vi "Protocol.Command.Main.vi"(8 "Error":errorcluster, 11 "J1939 Main Configuration":T1 {"Stream Refs"."Port Settings"."FD ISO Mode" items=["ISO", "Non ISO", "ISO Legacy"]; "Stream Refs"."Port Settings"."Termination" items=["Off", "On"]; "Stream Refs"."Port Settings"."Mode" items=["CAN 2.0", "CAN FD", "CAN FD+BRS"]}) -> (0 "error out":errorcluster)   [LabVIEW 2023, in "J1939 Addon Engine.lvlib"]
uses:
  J1939 Addon Engine.lvlib
  Types/Protocol.Configuration.ctl
  <vilib>/NI/NI VeriStand Addon Network Comm/Engine/VeriStand Comm.lvclass
  <vilib>/NI/NIVS Inline Async API/_VS Inline Async API/Process/Process.lvclass
  Types/Protocol.Refs.ctl
  Support Libraries/J1939 Utilities/Types/CAN Outgoing Message Cluster.ctl
  Types/Protocol.RQST Lookup Table Reference.ctl
  Types/Protocol.Address Table Reference.ctl
  Types/Protocol.XNET Settings.ctl
  <vilib>/NI/NIVS Inline Async API/_Data Access Engine/Data Access Engine/Types/Read.DVR.ctl
  <vilib>/NI/NIVS Inline Async API/_Data Access Engine/Access Type Classes/Read/Read.lvclass
  <vilib>/NI/NIVS Inline Async API/_Data Access Engine/Data Access Engine/Types/Write.DVR.ctl
  <vilib>/NI/NIVS Inline Async API/_Data Access Engine/Access Type Classes/Write/Write.lvclass
  Types/CounterAndProtectionFrames.ctl
  SubModules/Frame-Protection-Support/Source/Engine/Types/RT Frame Settings.ctl
  SubModules/Frame-Protection-Support/Source/Shared/Types/Exported Frame Type.ctl
  SubModules/Frame-Protection-Support/Source/Engine/Types/RT Protection Configuration.ctl
  SubModules/Frame-Protection-Support/Source/Shared/Types/Protection Type.ctl
  SubModules/Frame-Protection-Support/Source/Shared/Types/XNET Signal Configuration.ctl
  SubModules/Frame-Protection-Support/Source/Shared/Types/Exported Counter Settings.ctl
  SubModules/Frame-Protection-Support/Source/Shared/Types/Exported Event Trigger Type.ctl
  SubModules/CAN-Streaming-Support/Source/Addon/Addon Engine/Types/Engine Stream Refs.ctl
  SubModules/CAN-Streaming-Support/Source/Addon/Addon Shared/Types/Direction Filter.ctl
  SubModules/CAN-Streaming-Support/Source/Addon/Addon Shared/Types/Type Filter.ctl
  SubModules/CAN-Streaming-Support/Source/Addon/Addon Shared/Types/Filter Parameters.ctl
  SubModules/CAN-Streaming-Support/Source/Addon/Addon Engine/Types/Engine Stream Port Settings.ctl
  Types/Protocol.Command.Responses.ctl
  Types/Protocol.Command.Commands.ctl
  <vilib>/NI/NIVS Inline Async API/_Data Access Engine/Access Type Classes/Read/Read.lvclass/Read.ctl
  <vilib>/NI/NIVS Inline Async API/_Data Access Engine/Access Type Classes/Write/Write.lvclass/Write.ctl
  Addon Shared/Types/DTC_Action.ctl
  <vilib>/NI/NIVS Inline Async API/_VS Inline Async API/Process/Process.lvclass/Process.ctl
  <vilib>/NI/NIVS Inline Async API/_Data Access Engine/Data Access Engine/Methods/Write.Data.vi
  <vilib>/NI/NIVS Inline Async API/_Data Access Engine/Data Access Engine/Methods/Read.Data.vi
  <vilib>/NI/NIVS Inline Async API/_Data Access Engine/Access Type Classes/Write/Write.ProcessData.vi
  <vilib>/NI/NIVS Inline Async API/_VS Inline Async API/Error Handling Process/SubVIs/Error.ConvertArray.vi
  <vilib>/NI/NIVS Inline Async API/_Data Access Engine/Access Type Classes/Read/Read.ProcessData.vi
  <vilib>/NI/NIVS Inline Async API/_Data Access Engine/Access Type Classes/Write/Write.Buffer.vi
  <vilib>/NI/NIVS Inline Async API/_Data Access Engine/Access Type Classes/Write/Write.Commit.vi
  Addon Shared/J1939 Addon Shared.lvlib
  APIs/Host Automation API/J1939 Host Automation API.lvlib
  <vilib>/NI VeriStand/Custom Device Tools/Custom Device Utility Library/Custom Device Utility Library.lvlib
  <vilib>/NI/NIVS Inline Async API/_Data Access Engine/Data Access Engine/Data Access Engine.lvclass
  Support Libraries/J1939 Utilities/J1939 Utilities.lvlib
  SubModules/Frame-Protection-Support/Source/Engine/Protection and Counter Support Engine.lvlib
  SubModules/Frame-Protection-Support/Source/Shared/Protection and Counter Support Shared.lvlib
  SubModules/CAN-Streaming-Support/Source/Addon/Addon Shared/CAN Stream Support Shared.lvlib
  SubModules/CAN-Streaming-Support/Source/Addon/Addon Engine/CAN Stream Support Engine.lvlib
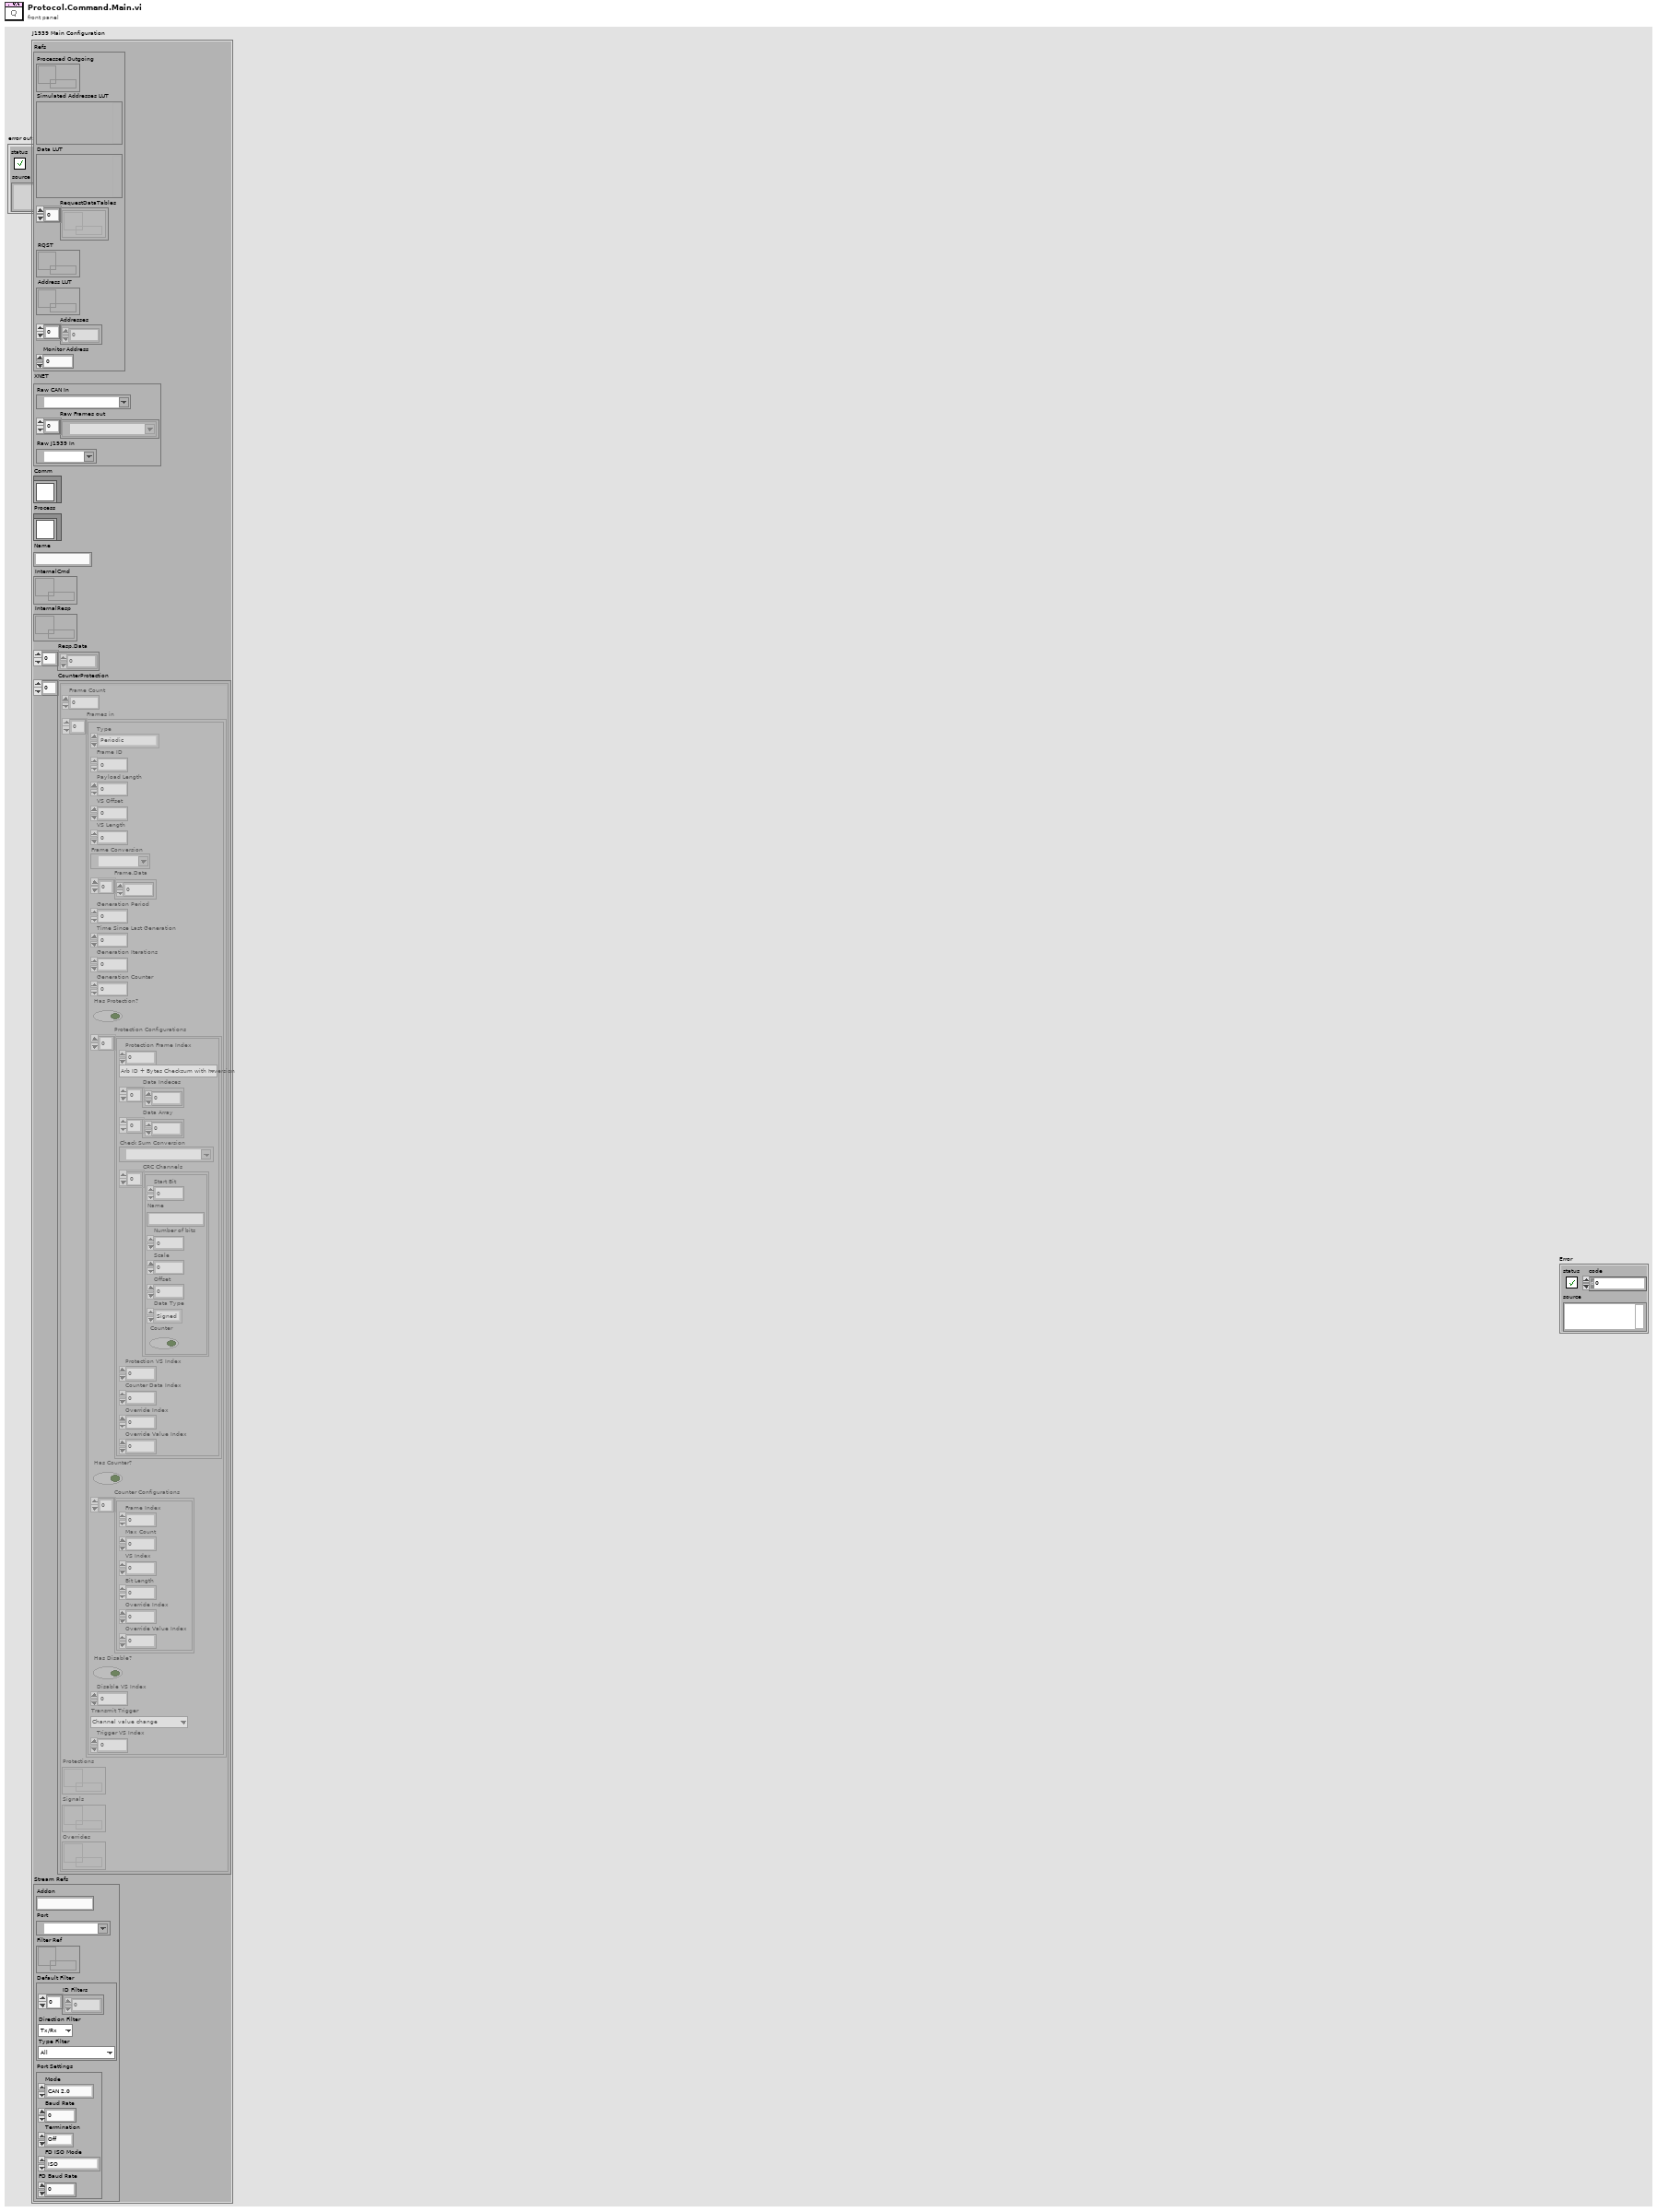
[diagram p1: front panel]
types:
  T1 = typedef "J1939 Addon Engine.lvlib/Protocol.Configuration.ctl" = cluster{"Refs":T2, "XNET":T5, "Comm":refnum<class "VeriStand Comm.lvclass">, "Process":refnum<class "Process.lvclass">, "Name":string, "InternalCmd":T6, "InternalResp":T7, "Resp.Data":dbl[], "CounterProtection":T8[], "Stream Refs":T16}
  T2 = typedef "J1939 Addon Engine.lvlib/Protocol.Refs.ctl" = cluster{"Processed Outgoing":refnum<queue>, "Simulated Addresses LUT":variant, "Data LUT":variant, "RequestDataTables":refnum<k33>[], "RQST":T3, "Address LUT":T4, "Addresses":u8[], "Monitor Address":u8}
  T3 = typedef "J1939 Addon Engine.lvlib/Protocol.RQST Lookup Table Reference.ctl" = refnum<data-value>
  T4 = typedef "J1939 Addon Engine.lvlib/Protocol.Address Table Reference.ctl" = refnum<data-value>
  T5 = typedef "J1939 Addon Engine.lvlib/Protocol.XNET Settings.ctl" = cluster{"Raw CAN In":refnum<k21>, "Raw Frames out":refnum<k21>[], "Raw J1939 In":refnum<k21>}
  T6 = typedef "Data Access Engine.lvlib/Data Access Engine.lvclass/Read.DVR.ctl" = refnum<data-value>
  T7 = typedef "Data Access Engine.lvlib/Data Access Engine.lvclass/Write.DVR.ctl" = refnum<data-value>
  T8 = typedef "J1939 Addon Engine.lvlib/CounterAndProtectionFrames.ctl" = cluster{"Frame Count":i32, "Frames in":T9[], "Protections":T7, "Signals":T6, "Overrides":T6}
  T9 = typedef "Protection and Counter Support Engine.lvlib/RT Frame Settings.ctl" = cluster{"Type":T10, "Frame ID":u32, "Payload Length":u32, "VS Offset":i32, "VS Length":i32, "Frame Conversion":refnum<k21>, "Frame.Data":dbl[], "Generation Period":u32, "Time Since Last Generation":u32, "Generation Iterations":u32, "Generation Counter":u32, "Has Protection?":bool, "Protection Configurations":T11[], "Has Counter?":bool, "Counter Configurations":T14[], "Has Disable?":bool, "Disable VS Index":i32, "Transmit Trigger":T15, "Trigger VS Index":i32}
  T10 = typedef "Protection and Counter Support Shared.lvlib/Exported Frame Type.ctl" = enum16{"Periodic", "Event", "Periodic/Event"}
  T11 = typedef "Protection and Counter Support Engine.lvlib/RT Protection Configuration.ctl" = cluster{"Protection Frame Index":i32, "Protection Type":T12, "Data Indeces":i32[], "Data Array":dbl[], "Check Sum Conversion":refnum<k21>, "CRC Channels":T13[], "Protection VS Index":i32, "Counter Data Index":i32, "Override Index":i32, "Override Value Index":i32}
  T12 = typedef "Protection and Counter Support Shared.lvlib/Protection Type.ctl" = enum16{"Arb ID + Bytes Checksum with Inversion", "Arb ID + Bytes CRC with Inversion", "Reversed Raw Signal Checksum with Inversion", "Concatenated Two's Compliment"}
  T13 = typedef "Protection and Counter Support Shared.lvlib/XNET Signal Configuration.ctl" = cluster{"Start Bit":i32, "Name":string, "Number of bits":i32, "Scale":dbl, "Offset":dbl, "Data Type":u32, "Counter":bool}
  T14 = typedef "Protection and Counter Support Shared.lvlib/Exported Counter Settings.ctl" = cluster{"Frame Index":i32, "Max Count":dbl, "VS Index":i32, "Bit Length":i64, "Override Index":i32, "Override Value Index":i32}
  T15 = typedef "Protection and Counter Support Shared.lvlib/Exported Event Trigger Type.ctl" = enum16{"Channel value change", "Trigger channel (not zero)", "Channel value change or trigger channel (not zero)", "Trigger channel (any value change)", "Channel value change or trigger channel (any value change)"}
  T16 = typedef "CAN Stream Support Engine.lvlib/Engine Stream Refs.ctl" = cluster{"Addon":string, "Port":refnum<k21>, "Filter Ref":refnum<data-value>, "Default Filter":T17, "Port Settings":T20}
  T17 = typedef "CAN Stream Support Shared.lvlib/Filter Parameters.ctl" = cluster{"ID Filters":u32[], "Direction Filter":T18, "Type Filter":T19}
  T18 = typedef "CAN Stream Support Shared.lvlib/Direction Filter.ctl" = enum16{"Tx/Rx", "Rx", "Tx"}
  T19 = typedef "CAN Stream Support Shared.lvlib/Type Filter.ctl" = enum16{"All", "CAN Data", "CAN Remote", "CAN Bus Error", "CAN 2.0 Data", "CAN FD Data", "CAN FD+BRS Data", "J1939 Data", "Delay", "Log Trigger", "Start Trigger"}
  T20 = typedef "CAN Stream Support Engine.lvlib/Engine Stream Port Settings.ctl" = cluster{"Mode":u32, "Baud Rate":u64, "Termination":u32, "FD ISO Mode":u32, "FD Baud Rate":u64}
  T21 = typedef "NI STM.lvlib/TCP Connection Info.ctl" = cluster{"connection ID":refnum<k5>, "meta data":T22[]}
  T22 = typedef "NI STM.lvlib/MetaDataElement.ctl" = string
  T23 = typedef "J1939 Addon Engine.lvlib/Protocol.Command.Responses.ctl" = enum16{"Diagnostic Error Code", "Diagnostic Command Success", "# of DTCs Found", "Request DTC Status"}
  T24 = typedef "J1939 Addon Engine.lvlib/Protocol.Command.Commands.ctl" = enum16{"Diagnostic Command", "Expected DTC", "Address to Query", "DTC Clear Type"}
  T25 = typedef "J1939 Addon Shared.lvlib/DTC_Action.ctl" = enum16{"ALL", "ACTIVE", "INACTIVE"}
  T26 = typedef "J1939 Addon Engine.lvlib/Protocol.Command.States.ctl" = enum8{"Idle", "Refresh Address", "Verify DTCs", "Clear DTCs", "Clear Status Bit", "Clear Error Bit"}
  T27 = typedef "J1939 Addon Shared.lvlib/Verify DTC_Status.ctl" = enum16{"NOT_PRESENT", "ACTIVE", "INACTIVE"}
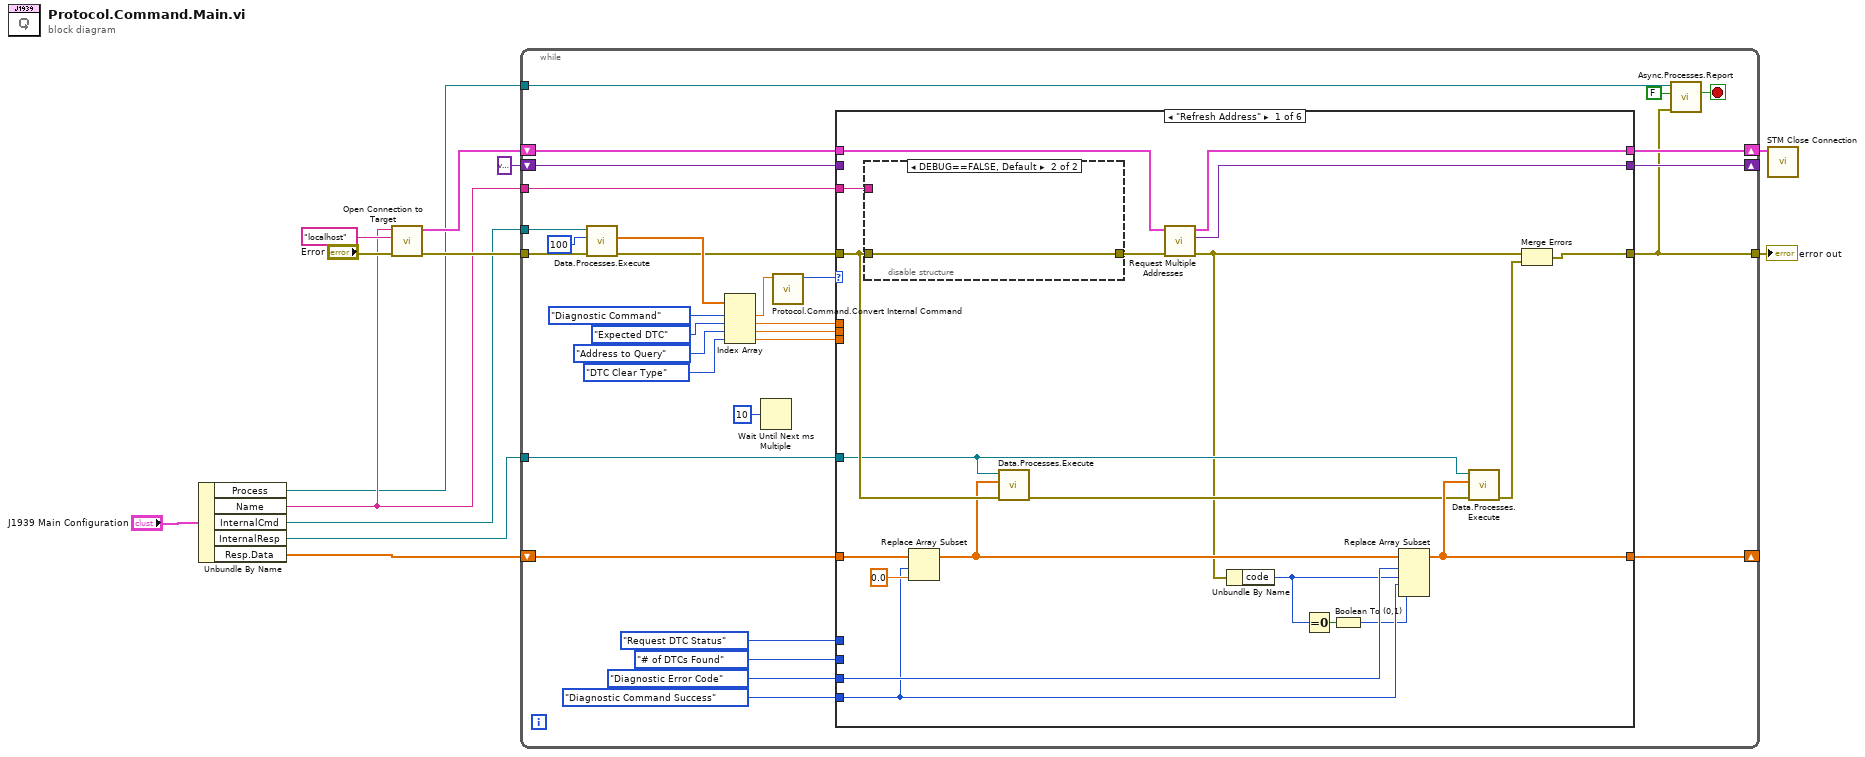
[diagram p0: block diagram]
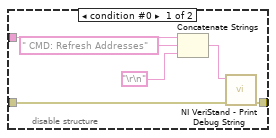
[diagram p2: hidden frame]
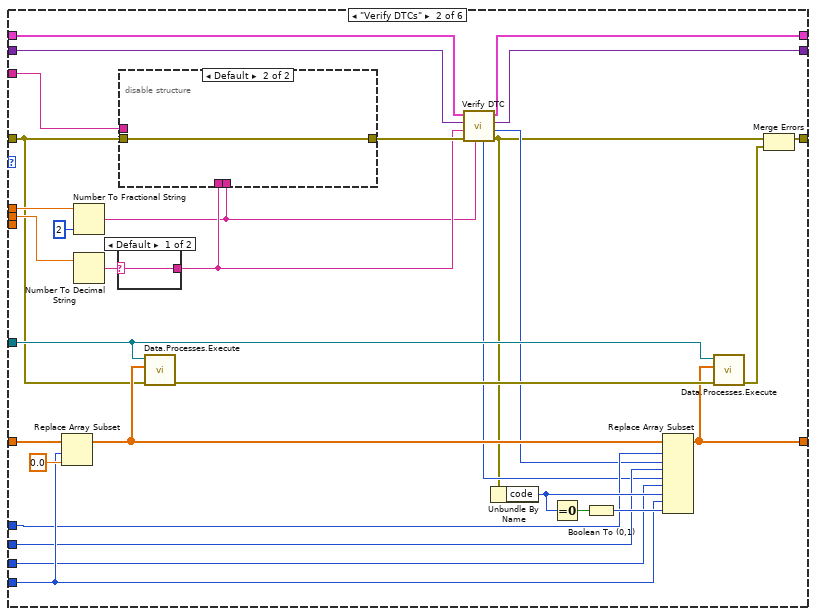
[diagram p3: hidden frame]
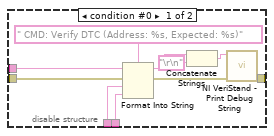
[diagram p4: hidden frame]
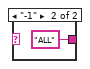
[diagram p5: hidden frame]
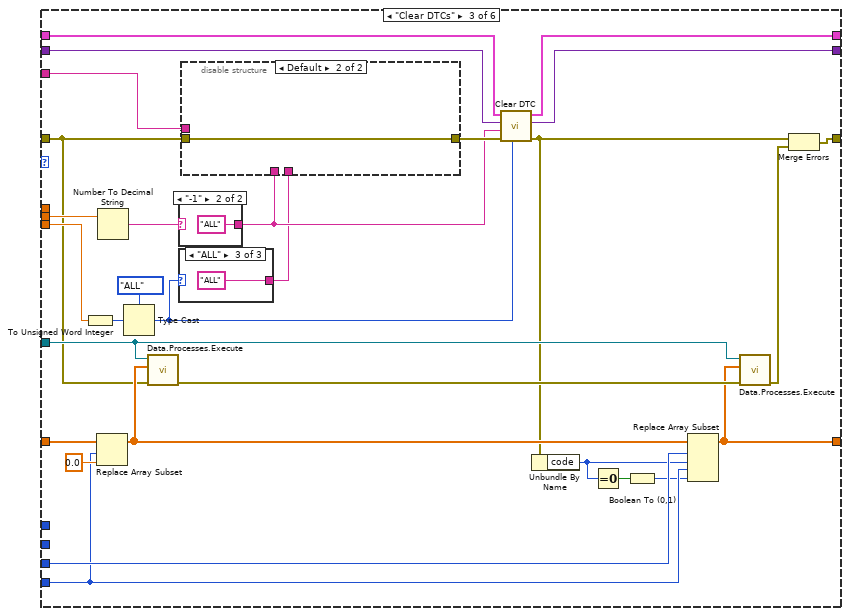
[diagram p6: hidden frame]
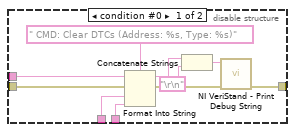
[diagram p7: hidden frame]
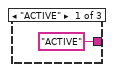
[diagram p8: hidden frame]
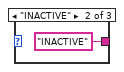
[diagram p9: hidden frame]
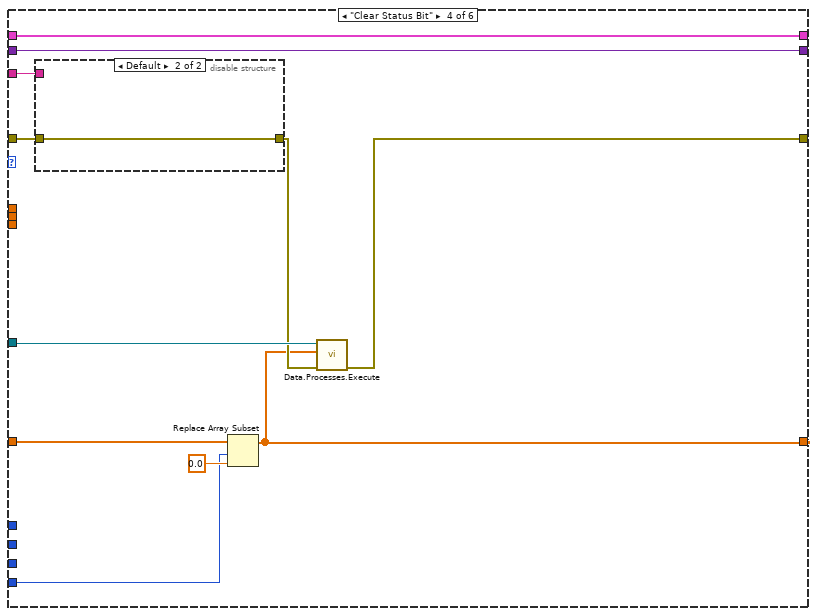
[diagram p11: hidden frame]
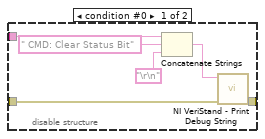
[diagram p12: hidden frame]
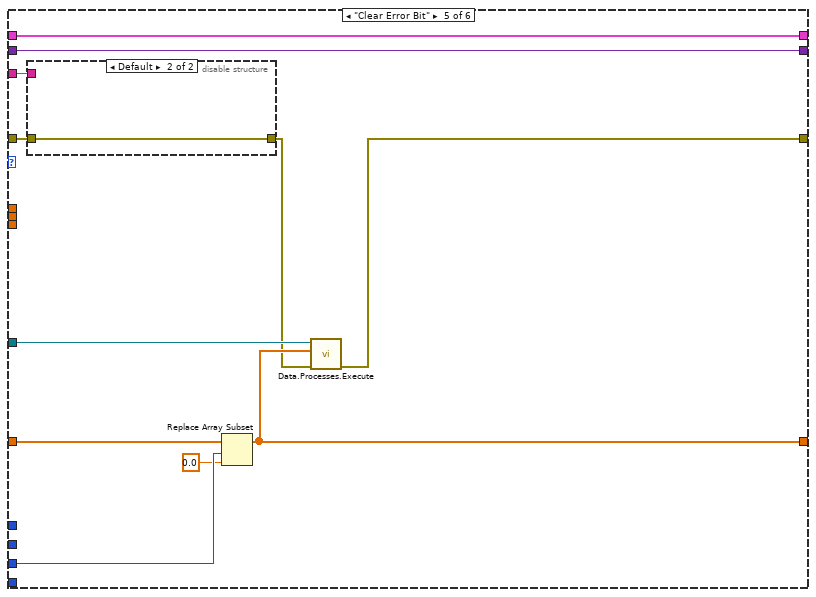
[diagram p13: hidden frame]
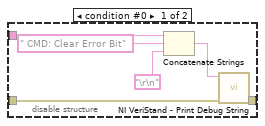
[diagram p14: hidden frame]
diagram:
  n1 = Unbundle By Name("J1939 Main Configuration") -> ("Process"=w3:refnum<class "Process.lvclass">, "Name"=w4:string, "InternalCmd"=w5:T6, "InternalResp"=w6:T7, "Resp.Data"=w1:dbl[])
  n2 = call "Open Connection to Target.vi"("error in (no error)"="Error", "IP Address"="localhost", "TCP Service"=w4) -> ("error out"=w9:errorcluster, "connection info"=w12:T21)  [unwired: 7 in]
  n3 = while {
    shift-right: [w43] -> _
    shift-left: variant ("Address Lookup Table Out") -> [w42]
    shift-right: [w41] -> w10
    shift-left: w12 -> [w44]
    tunnel: [w34] -> w8
    tunnel: w9 -> [w32]
    tunnel: w3 -> [w38]
    tunnel: w4 -> [w37]
    tunnel: w5 -> [w24]
    shift-right: [w17] -> _
    shift-left: w1 -> [w18]
    tunnel: w6 -> [w19]
    stop <- w39 stop-if-true
    n4 = call-poly <vilib>:"Data.Processes.Execute.vi"("error in (no error)"=w32, "timeout ms"=100 ("timeout in ms (0)"), "Ref"=w24) -> ("error out"=w25:errorcluster, "Values"=w31:dbl[])  [unwired: 6 in, 1 out]
    n5 = Index Array(array=w31, index #1=Protocol.Command.Commands."Diagnostic Command" ("Enum"), index #2=Protocol.Command.Commands."Expected DTC" ("Enum"), index #3=Protocol.Command.Commands."Address to Query" ("Enum"), index #4=Protocol.Command.Commands."DTC Clear Type" ("Enum")) -> (element #1=w26:dbl, element #2=w16:dbl, element #3=w15:dbl, element #4=w14:dbl)
    n6 = Wait Until Next ms Multiple(millisecond multiple=u32 10) -> ()  [unwired: 1 out]
    n7 = call "Protocol.Command.Convert Internal Command.vi"("Value"=w26) -> ("Enum"=w35:T26)  [unwired: 9 in, 1 out]
    n8 = case shown="\"Refresh Address\"" w35 {
      tunnel: w44 -> [w64 w102 w144 w171 w189 w199]
      tunnel: [w63 w100 w142 w170 w188 w198] -> w43
      tunnel: w42 -> [_ w101 w143 w170 w188 w198]
      tunnel: [w62 w99 w141 w171 w189 w199] -> w41
      tunnel: w25 -> [w59 w84 w116 w169 w187 w200]
      tunnel: [w45 w72 w120 w163 w180 w200] -> w34
      tunnel: w37 -> [w51 w93 w133 w162 w179 _]
      tunnel: Protocol.Command.Responses."Request DTC Status" ("Enum 2") -> [_ w78 _ _ _ _]
      tunnel: Protocol.Command.Responses."# of DTCs Found" ("Enum 2") -> [_ w79 _ _ _ _]
      tunnel: Protocol.Command.Responses."Diagnostic Error Code" ("Enum 2") -> [w56 w80 w126 _ w184 _]
      tunnel: Protocol.Command.Responses."Diagnostic Command Success" ("Enum 2") -> [w55 w81 w125 w165 _ _]
      tunnel: w19 -> [w50 w87 w128 w167 w186 _]
      tunnel: w18 -> [w58 w88 w127 w166 w185 w197]
      tunnel: [w49 w73 w117 w161 w182 w197] -> w17
      tunnel: w16 -> [_ w86 _ _ _ _]
      tunnel: w15 -> [_ w85 w118 _ _ _]
      tunnel: w14 -> [_ _ w119 _ _ _]
      frame "Refresh Address" {
        n9 = disable-structure shown="DEBUG==FALSE, Default" {
          disable-tunnel: w59 -> [w67 w71]
          disable-tunnel: [w66 w71] -> w52
          disable-tunnel: w51 -> [w65 _]
          frame condition #0 {
            n10 = Concatenate Strings(w65, " CMD: Refresh Addresses" ("string"), "\r\n") -> (w69:string)
            n11 = call <vilib>:"NI VeriStand - Print Debug String.vi"("error in (no error)"=w67, "Message"=w69) -> ("error out"=w66:errorcluster)  [unwired: 9 in]
          }
          frame condition #1 (active) {
          }
        }
        n12 = Replace Array Subset(array=w58, new element=0.0 ("Value"), index=w55) -> (w57:dbl[])
        n13 = call-poly <vilib>:"Data.Processes.Execute.vi"("error in (no error)"=w59, "Values"=w57, "Ref"=w50) -> ("error out"=w48:errorcluster)  [unwired: 8 in]
        n14 = call "Request Multiple Addresses.vi"("error in (no error)"=w52, "connection info"=w64) -> ("error out"=w47:errorcluster, "variant"=w63:variant, "connection info"=w62:T21)  [unwired: 6 in, 1 out]
        n15 = Unbundle By Name(w47) -> ("code"=w53:i32)
        n16 = Equal To 0?(x=w53) -> (x = 0?=w61:bool)
        n17 = Boolean To (0,1)(Boolean=w61) -> (0, 1=w54:i16)
        n18 = Replace Array Subset(array=w57, new element #1=w53, index #1=w56, new element #2=w54, index #2=w55) -> (w49:dbl[])
        n19 = call-poly <vilib>:"Data.Processes.Execute.vi"("error in (no error)"=w48, "Values"=w49, "Ref"=w50) -> ("error out"=w46:errorcluster)  [unwired: 8 in]
        n20 = Merge Errors(w47, w46) -> (w45:errorcluster)
      }
      frame "Verify DTCs" {
        n21 = Replace Array Subset(array=w88, new element=0.0 ("Value"), index=w81) -> (w90:dbl[])
        n22 = Number To Fractional String(number=w86, precision (6)=i16 2) -> (F-format string=w94:string)  [unwired: 2 in]
        n23 = Number To Decimal String(number=w85) -> (decimal integer string=w98:string)  [unwired: 1 in]
        n24 = case shown="Default" w98 {
          selector: w98 -> [w114 _]
          tunnel: [w114 "ALL"] -> w95
          frame Default {
          }
          frame "-1" {
          }
        }
        n25 = disable-structure shown="Default" {
          disable-tunnel: [w109 w113] -> w96
          disable-tunnel: w95 -> [w108 _]
          disable-tunnel: w94 -> [w107 _]
          disable-tunnel: w93 -> [w104 _]
          disable-tunnel: w84 -> [w103 w113]
          frame condition #0 {
            n26 = Format Into String(format string=" CMD: Verify DTC (Address: %s, Expected: %s)" ("string"), initial string=w104, error in=w103, w108, w107) -> (resulting string=w111:string, error out=w110:errorcluster)
            n27 = Concatenate Strings(w111, "\r\n") -> (w106:string)
            n28 = call <vilib>:"NI VeriStand - Print Debug String.vi"("error in (no error)"=w110, "Message"=w106) -> ("error out"=w109:errorcluster)  [unwired: 9 in]
          }
          frame condition #1 (active) {
          }
        }
        n29 = call-poly <vilib>:"Data.Processes.Execute.vi"("error in (no error)"=w84, "Values"=w90, "Ref"=w87) -> ("error out"=w89:errorcluster)  [unwired: 8 in]
        n30 = call "Verify DTC.vi"("Expected DTC"=w94, "error in"=w96, "Address"=w95, "Address Lookup Table"=w101, "connection info"=w102) -> ("error out"=w75:errorcluster, "Status"=w77:T27, "Address Lookup Table Out"=w100:variant, "connection info"=w99:T21, "Found DTCs"=w76:i32)  [unwired: 2 in]
        n31 = Unbundle By Name(w75) -> ("code"=w82:i32)
        n32 = Equal To 0?(x=w82) -> (x = 0?=w92:bool)
        n33 = Boolean To (0,1)(Boolean=w92) -> (0, 1=w83:i16)
        n34 = Replace Array Subset(array=w90, new element #1=w77, index #1=w78, new element #2=w76, index #2=w79, new element #3=w82, index #3=w80, new element #4=w83, index #4=w81) -> (w73:dbl[])
        n35 = call-poly <vilib>:"Data.Processes.Execute.vi"("error in (no error)"=w89, "Values"=w73, "Ref"=w87) -> ("error out"=w74:errorcluster)  [unwired: 8 in]
        n36 = Merge Errors(w75, w74) -> (w72:errorcluster)
      }
      frame "Clear DTCs" {
        n37 = To Unsigned Word Integer(number=w119) -> (unsigned 16bit integer=w139:u16)
        n38 = Replace Array Subset(array=w127, new element=0.0 ("Value"), index=w125) -> (w130:dbl[])
        n39 = Number To Decimal String(number=w118) -> (decimal integer string=w140:string)  [unwired: 1 in]
        n40 = Type Cast(type=DTC_Action."ALL" ("Action"), x=w139) -> (*(type *) &x=w137:T25)
        n41 = call-poly <vilib>:"Data.Processes.Execute.vi"("error in (no error)"=w116, "Values"=w130, "Ref"=w128) -> ("error out"=w129:errorcluster)  [unwired: 8 in]
        n42 = case shown="\"-1\"" w140 {
          selector: w140 -> [w159 _]
          tunnel: [w159 "ALL"] -> w135
          frame Default {
          }
          frame "-1" {
          }
        }
        n43 = case shown="\"ALL\"" w137 {
          tunnel: ["ACTIVE" "INACTIVE" "ALL"] -> w134
          frame "ACTIVE" {
          }
          frame "INACTIVE" {
          }
          frame "ALL" {
          }
        }
        n44 = disable-structure shown="Default" {
          disable-tunnel: [w152 w155] -> w136
          disable-tunnel: w135 -> [w151 _]
          disable-tunnel: w134 -> [w150 _]
          disable-tunnel: w133 -> [w146 _]
          disable-tunnel: w116 -> [w145 w155]
          frame condition #0 {
            n45 = Format Into String(format string=" CMD: Clear DTCs (Address: %s, Type: %s)" ("string"), initial string=w146, error in=w145, w151, w150) -> (resulting string=w148:string, error out=w153:errorcluster)
            n46 = Concatenate Strings(w148, "\r\n") -> (w147:string)
            n47 = call <vilib>:"NI VeriStand - Print Debug String.vi"("error in (no error)"=w153, "Message"=w147) -> ("error out"=w152:errorcluster)  [unwired: 9 in]
          }
          frame condition #1 (active) {
          }
        }
        n48 = call "Clear DTC.vi"("Action"=w137, "error in"=w136, "Address (ALL)"=w135, "Address Lookup Table"=w143, "connection info"=w144) -> ("error out"=w121:errorcluster, "Address Lookup Table Out"=w142:variant, "connection info"=w141:T21)  [unwired: 4 in]
        n49 = Unbundle By Name(w121) -> ("code"=w123:i32)
        n50 = Equal To 0?(x=w123) -> (x = 0?=w132:bool)
        n51 = Boolean To (0,1)(Boolean=w132) -> (0, 1=w124:i16)
        n52 = Replace Array Subset(array=w130, new element #1=w123, index #1=w126, new element #2=w124, index #2=w125) -> (w117:dbl[])
        n53 = call-poly <vilib>:"Data.Processes.Execute.vi"("error in (no error)"=w129, "Values"=w117, "Ref"=w128) -> ("error out"=w122:errorcluster)  [unwired: 8 in]
        n54 = Merge Errors(w121, w122) -> (w120:errorcluster)
      }
      frame "Clear Status Bit" {
        n55 = disable-structure shown="Default" {
          disable-tunnel: w169 -> [w177 w178]
          disable-tunnel: [w173 w178] -> w164
          disable-tunnel: w162 -> [w172 _]
          frame condition #0 {
            n56 = Concatenate Strings(w172, " CMD: Clear Status Bit" ("string"), "\r\n") -> (w175:string)
            n57 = call <vilib>:"NI VeriStand - Print Debug String.vi"("error in (no error)"=w177, "Message"=w175) -> ("error out"=w173:errorcluster)  [unwired: 9 in]
          }
          frame condition #1 (active) {
          }
        }
        n58 = Replace Array Subset(array=w166, new element=0.0 ("Value"), index=w165) -> (w161:dbl[])
        n59 = call-poly <vilib>:"Data.Processes.Execute.vi"("error in (no error)"=w164, "Values"=w161, "Ref"=w167) -> ("error out"=w163:errorcluster)  [unwired: 8 in]
      }
      frame "Clear Error Bit" {
        n60 = disable-structure shown="Default" {
          disable-tunnel: w187 -> [w195 w196]
          disable-tunnel: [w191 w196] -> w181
          disable-tunnel: w179 -> [w190 _]
          frame condition #0 {
            n61 = Concatenate Strings(w190, " CMD: Clear Error Bit" ("string"), "\r\n") -> (w193:string)
            n62 = call <vilib>:"NI VeriStand - Print Debug String.vi"("error in (no error)"=w195, "Message"=w193) -> ("error out"=w191:errorcluster)  [unwired: 9 in]
          }
          frame condition #1 (active) {
          }
        }
        n63 = Replace Array Subset(array=w185, new element=0.0 ("Value"), index=w184) -> (w182:dbl[])
        n64 = call-poly <vilib>:"Data.Processes.Execute.vi"("error in (no error)"=w181, "Values"=w182, "Ref"=w186) -> ("error out"=w180:errorcluster)  [unwired: 8 in]
      }
      frame "Idle" {
      }
    }
    n65 = call <vilib>:"Async.Processes.Report.vi"("Error"=w34, "Stop Async on Error?"=FALSE ("Stop on Error?"), "Process in"=w38) -> ("Stop"=w39:bool)  [unwired: 7 in, 1 out]
  }
  "error out" <- w8
  n66 = call "STM Close Connection.vi"("connection info"=w10) -> ()  [unwired: 10 in, 1 out]
